vi "UDP Add Remove Last Update Channel.vi"(8 "error in (no error)":errorcluster, 10 "Last Update Tag?":bool, 11 "node References":T1) -> (0 "error out":errorcluster, 3 "node References out":T1)   [LabVIEW 2015, in "E2E Tag Exchange editor node.lvclass"]
uses:
  E2E Tag Exchange editor node.lvclass
  object references.ctl
  <vilib>/NI/DCAF/Tag Editor Core/Configuration Editor/Classes/Engine Parent/Engine Parent Editor Node.lvclass
  <vilib>/NI/Tag Bus Module Framework/channel/TBM channel.lvclass
  <vilib>/NI/Tag Bus/tag/Data Type.ctl
  <vilib>/NI/Tag Bus Module Framework/channel/channel classification.ctl
  <vilib>/NI/Tag Bus/tag/tag descriptor.lvclass
  <vilib>/NI/Module Execution Interface/Engine Configuration/engine configuration.lvclass
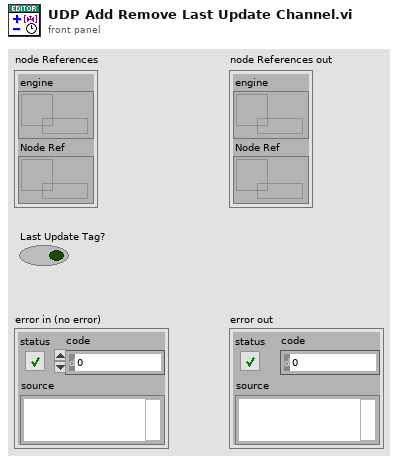
[diagram p1: front panel]
types:
  T1 = typedef "E2E Tag Exchange editor node.lvclass/object references.ctl" = cluster{"engine":refnum<data-value>, "Node Ref":refnum<data-value>}
  T2 = typedef "TBM channel.lvclass/channel classification.ctl" = enum16{"input data", "output data", "processing parameter", "processing result"}
  T3 = typedef "tag bus.lvlib/tag descriptor.lvclass/Data Type.ctl" = enum16{"Double", "Single", "I64", "I32", "I16", "I8", "U64", "U32", "U16", "U8", "Boolean", "String", "Array of Double", "Array of Single", "Array of I64", "Array of I32", "Array of I16", "Array of I8", "Array of U64", "Array of U32", "Array of U16", "Array of U8", "Array of Boolean", "Array of String"}
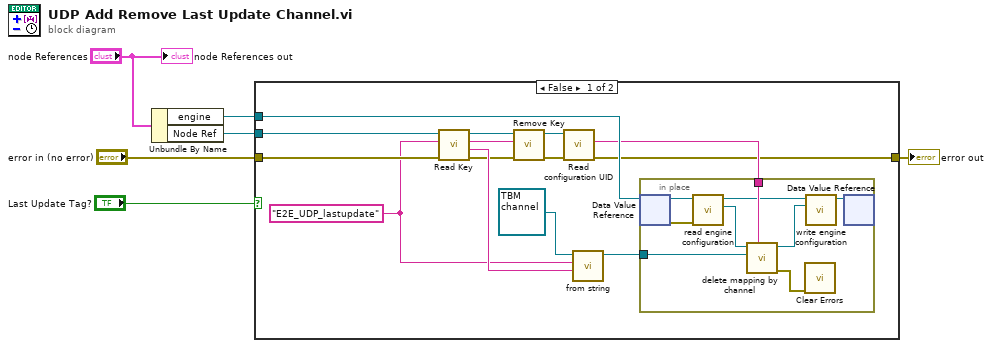
[diagram p0: block diagram]
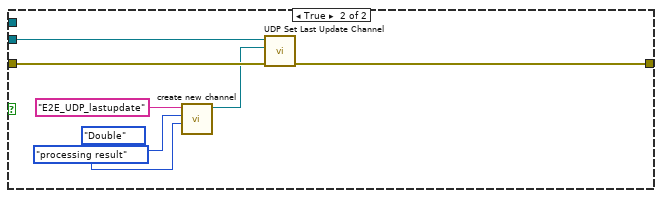
[diagram p2: hidden frame]
diagram:
  n1 = Unbundle By Name("node References") -> ("engine"=w1:refnum<data-value>, "Node Ref"=w5:refnum<data-value>)
  n2 = case shown="False" "Last Update Tag?" {
    tunnel: w5 -> [w19 w30]
    tunnel: "error in (no error)" -> [w15 w32]
    tunnel: [w7 w31] -> w2
    tunnel: w1 -> [w12 _]
    frame False {
      w13 = "E2E_UDP_lastupdate" ("Key")
      n3 = call "Read Key.vi"("error in (no error)"=w15, "Key"=w13, "E2E editor node in"=w19) -> ("error out"=w14:errorcluster, "Value"=w17:string, "E2E editor node out"=w18:refnum<data-value>)  [unwired: 6 in]
      n4 = call "Remove Key.vi"("error in (no error)"=w14, "Key"=w13, "E2E editor node in"=w18) -> ("error out"=w11:errorcluster, "E2E editor node out"=w10:refnum<data-value>)  [unwired: 7 in]
      n5 = call "Read configuration UID.vi"("error in (no error)"=w11, "E2E editor node in"=w10) -> ("error out"=w7:errorcluster, "Module UID"=w9:string)  [unwired: 7 in, 1 out]
      n6 = call-dynamic "from string.vi"("channel data"=w17, "identifier"=w13, "channel in"=refnum<class "TBM channel.lvclass"> refnum) -> ("channel out"=w8:refnum<class "TBM channel.lvclass">)  [unwired: 7 in, 1 out]
      n7 = in-place {
        in-place-border: w9 -> [w26]
        in-place-border: w8 -> [w24]
        n8 = in-place-dvr #1(w12) -> (w28:refnum<class "Engine Parent Editor Node.lvclass">, w27:errorcluster)
        n9 = call <vilib>:"read engine configuration.vi"("error in"=w27, "Engine Parent Editor Node in"=w28) -> ("engine configuration"=w25:refnum<class "engine configuration.lvclass">, "Engine Parent Editor Node out"=w21:refnum<class "Engine Parent Editor Node.lvclass">)  [unwired: 7 in, 1 out]
        n10 = call <vilib>:"delete mapping by channel.vi"("owner ID"=w26, "channel"=w24, "engine configuration in"=w25) -> ("error out"=w20:errorcluster, "engine configuration out"=w22:refnum<class "engine configuration.lvclass">)  [unwired: 7 in]
        n11 = call <vilib>:"Clear Errors.vi"("error in (no error)"=w20) -> ()  [unwired: 5 in, 2 out]
        n12 = call <vilib>:"write engine configuration.vi"("engine configuration"=w22, "Engine Parent Editor Node in"=w21) -> ("Engine Parent Editor Node out"=w23:refnum<class "Engine Parent Editor Node.lvclass">)  [unwired: 8 in, 1 out]
        n13 = in-place-dvr #1(w23) -> ()  [unwired: 2 out]
      }
    }
    frame True {
      n14 = call <vilib>:"create new channel.vi"("channel classification"=channel_classification."processing result", "data type"=Data_Type."Double", "channel name"="E2E_UDP_lastupdate" ("Key")) -> ("channel"=w29:refnum<class "TBM channel.lvclass">)  [unwired: 8 in]
      n15 = call "UDP Set Last Update Channel.vi"("error in (no error)"=w32, "TBM channel in"=w29, "Node Ref"=w30) -> ("error out"=w31:errorcluster)  [unwired: 7 in, 1 out]
    }
  }
  "error out" <- w2
  "node References out" <- "node References"
